vi "Write Pressure _10.vi"(8 "error in (no error)":errorcluster, 10 "Pressure *10":i64=70, 11 "CAD Dispense in":refnum<class "CAD Dispense.lvclass">) -> (0 "error out":errorcluster, 3 "CAD Dispense out":refnum<class "CAD Dispense.lvclass">)   [LabVIEW 2020, in "CAD Dispense.lvclass"]
uses:
  CAD Dispense.lvclass
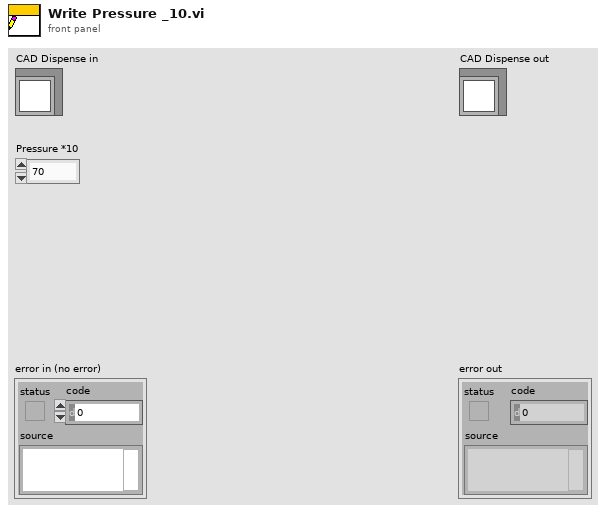
[diagram p1: front panel]
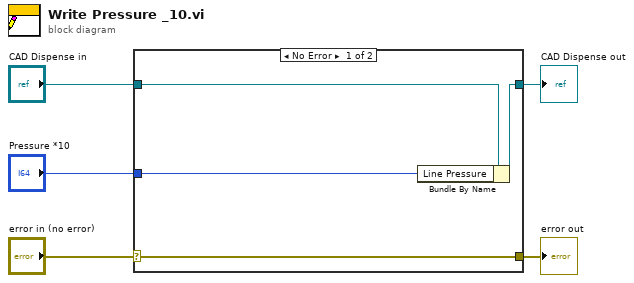
[diagram p0: block diagram]
diagram:
  n1 = case shown="No Error" "error in (no error)" {
    selector: "error in (no error)" -> [w9 w10]
    tunnel: [w9 w10] -> w4
    tunnel: [w7 w11] -> w2
    tunnel: "CAD Dispense in" -> [w8 w11]
    tunnel: "Pressure *10" -> [w6 _]
    frame No Error {
      n2 = Bundle By Name(cluster=w8, "Line Pressure"=w6) -> (w7:refnum<class "CAD Dispense.lvclass">)
    }
    frame Error {
    }
  }
  "error out" <- w4
  "CAD Dispense out" <- w2
